vi "Smoothing_Alignment_v12 (SubVI).vi"(0 "X center":dbl, 1 "Intensity Graph":dbl[][](array[numeric]), 5 "Y center":dbl, 7 "Mesh":dbl, 9 "X Scan Range":dbl, 11 "Y Scan Range":dbl, 12 "Z":dbl, 14 "System no.":i32, 15 "error in (no error)":errorcluster) -> (4 "Alignment Graph":dbl[][](array[numeric]), 10 "error out":errorcluster)   [LabVIEW 2023]
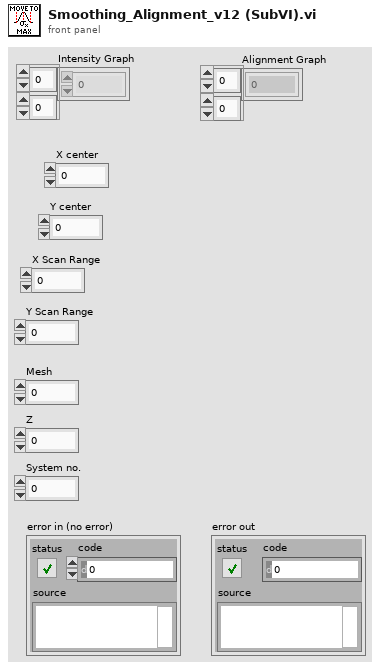
[diagram p1: front panel]
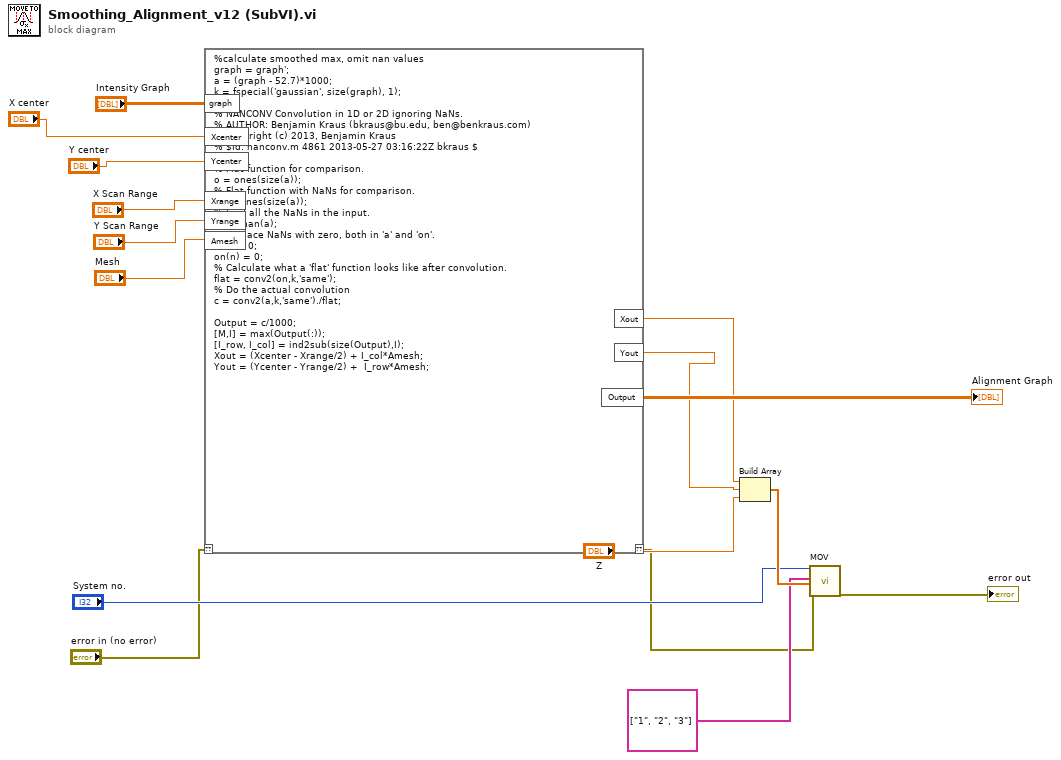
[diagram p0: block diagram]
diagram:
  n1 = script code="%calculate smoothed max, omit nan values\ngraph = graph';\na = (graph - 52.7)*1000;\nk = fspecial('gaussian', size(graph), 1);\n\n% NANCONV Convolution in 1D or 2D ignoring NaNs.\n% AUTHOR: Benjamin Kraus (bkraus@bu.edu, ben@benkraus.com)\n% Copyright (c) 2013, Benjamin Kraus\n% $Id: nanconv.m 4861 2013-05-27 03:16:22Z bkraus $\n\n% Flat function for comparison.\no = ones(size(a));\n% Flat function with NaNs for comparison.\non = ones(size(a));\n% Find all the NaNs in the input.\nn = isnan(a);\n% Replace NaNs with zero, both in 'a' and 'on'.\na(n) = 0;\non(n) = 0;\n% Calculate what a 'flat' function looks like after convolution.\nflat = conv2(on,k,'same');\n% Do the actual convolution\nc = conv2(a,k,'same')./flat;\n\nOutput = c/1000;\n[M,I] = max(Output(:));\n[I_row, I_col] = ind2sub(size(Output),I);\nXout = (Xcenter - Xrange/2) + I_col*Amesh;\nYout = (Ycenter - Yrange/2) +  I_row*Amesh;"("??"="error in (no error)", "graph"="Intensity Graph", "Xcenter"="X center", "Ycenter"="Y center", "Xrange"="X Scan Range", "Yrange"="Y Scan Range", "Amesh"="Mesh") -> ("??"=w5:errorcluster, "Xout"=w2:dbl, "Yout"=w4:dbl, "Output"=→"Alignment Graph":dbl[][])
  n2 = Build Array(w2, w4, "Z") -> (w16:dbl[])
  n3 = call "MOV.vi"("System no."="System no.", "Axes to move"=string[] ["1", "2", "3"], "Position values"=w16, "error in"=w5) -> ("error out"=→"error out":errorcluster)  [unwired: 1 in, 14 out]
